vi "stations Template Keys.vi"(7 "Station ID (\"\")":string, 8 "error in (no error)":errorcluster, 9 "Copy? (f)":bool, 10 "Edit? (f)":bool, 11 "Connection Refnum":T1) -> (0 "error out":errorcluster, 1 "Template Keys":T2, 3 "Connection Refnum":T1)   [LabVIEW 2011]
uses:
  ITK EXT/utils/keyedarr.llb/Keyed Array.ctl
  Summitek EXT/ODBC/SQL Controls/Connection Refnum.ctl
  server/database/Drivers/Driver Table Fields.ctl
  ITK EXT/utils/strutil.llb/Case Matching.ctl
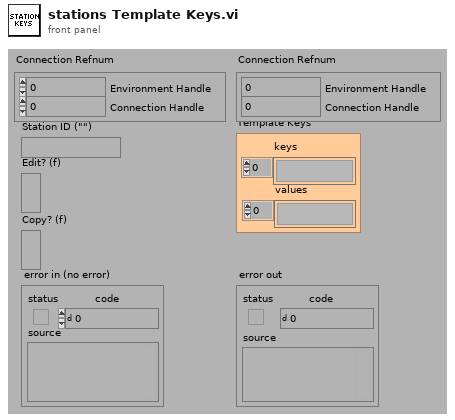
[diagram p1: front panel]
types:
  T1 = typedef "Connection Refnum.ctl" = cluster{"Environment Handle":i32, "Connection Handle":i32}
  T2 = typedef "Keyed Array.ctl" = cluster{"keys":string[], "values":string[]}
  T3 = typedef "Driver Table Fields.ctl" = enum16{"sxDriverId", "sType", "sVersion", "ixDriver"}
  T4 = typedef "Instrument Record.ctl" = cluster{"ixInstrument":i32, "sxInstrumentId":string, "sDriverId":string, "sDriverType":string, "sSerialNumber":string, "tLastCalibration":timestamp, "tCalibrationDue":timestamp, "sConfiguration":string}
  T5 = typedef "Station Record.ctl" = cluster{"ixStation":i32, "sxStationId":string, "sIP":string, "fVerified":bool}
  T6 = typedef "Driver Record.ctl" = cluster{"ixDriver":i32, "sxDriverId":string, "sType":string, "sVersion":string}
  T7 = typedef "Case Matching.ctl" = enum16{"a != A", "a == A", "system"}
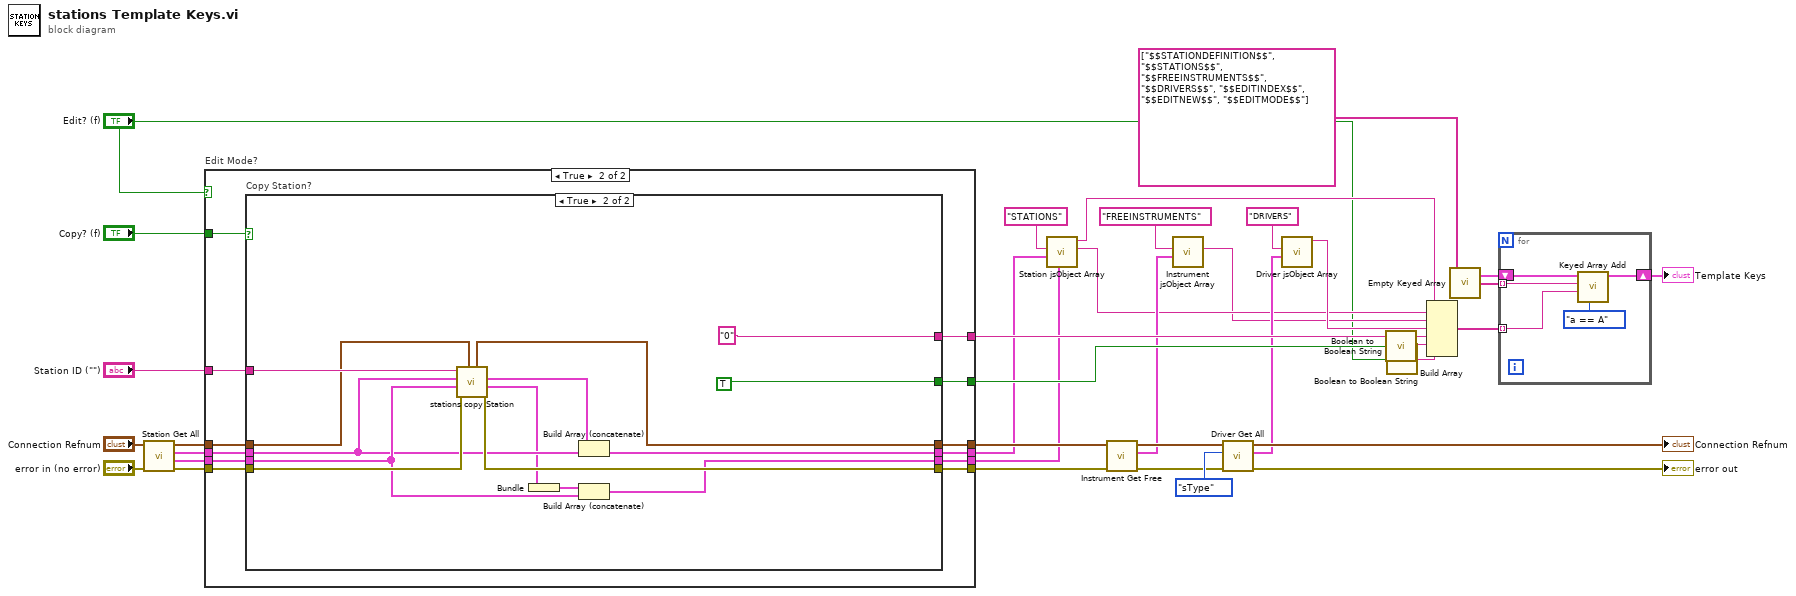
[diagram p0: block diagram]
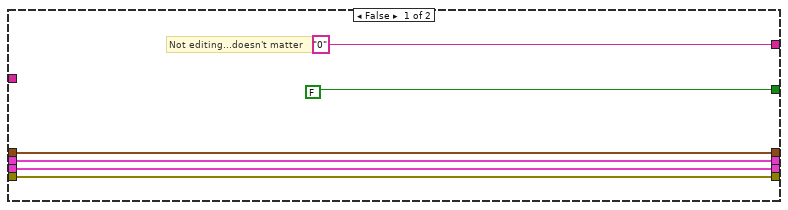
[diagram p2: hidden frame]
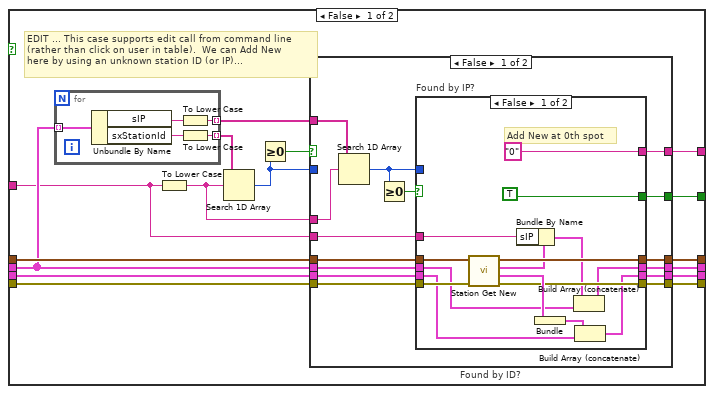
[diagram p3: hidden frame]
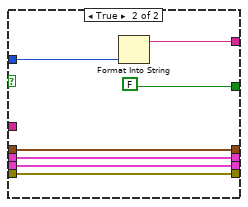
[diagram p4: hidden frame]
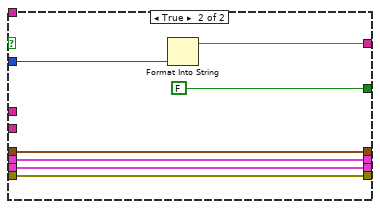
[diagram p5: hidden frame]
diagram:
  n1 = call "Station Get All.vi"("error in (no error)"="error in (no error)", "Connection Refnum"="Connection Refnum") -> ("error out"=w27:errorcluster, "All Station Instruments"=w22:cluster{"Instruments":T4[]}[], "Station Records"=w23:T5[], "Connection Refnum"=w24:T1)  [unwired: 2 in, 4 out]
  n2 = case "Edit Mode?" shown="True" "Edit? (f)" {
    tunnel: w23 -> [w41 w53]
    tunnel: [w41 w42] -> w13
    tunnel: w27 -> [w40 w52]
    tunnel: [w40 w51] -> w17
    tunnel: ["0" w50] -> w21
    tunnel: "Station ID (\"\")" -> [_ w49]
    tunnel: [FALSE w48] -> w19
    tunnel: "Copy? (f)" -> [_ w47]
    tunnel: w24 -> [w37 w44]
    tunnel: w22 -> [w38 w46]
    tunnel: [w38 w45] -> w12
    tunnel: [w37 w43] -> w15
    frame False {
      # "Not editing...doesn't matter"
    }
    frame True {
      n3 = case "Copy Station?" shown="True" w47 {
        tunnel: w49 -> [w54 w127]
        tunnel: w53 -> [w58 w123]
        tunnel: [w67 "0"] -> w50
        tunnel: [w66 w129] -> w51
        tunnel: w52 -> [w65 w130]
        tunnel: [w64 TRUE] -> w48
        tunnel: [w56 w128] -> w42
        tunnel: w46 -> [w57 w126]
        tunnel: [w55 w121] -> w45
        tunnel: w44 -> [w60 w120]
        tunnel: [w59 w119] -> w43
        frame False {
          # "EDIT ... This case supports edit call from command line\n(rather than click on user in table).  We can Add New\nhere by using an unknown station ID (or IP)..."
          n4 = for {
            tunnel: [w118] -> w69 mode=indexing
            tunnel: w58 -> [w117] mode=indexing
            tunnel: [w114] -> w62 mode=indexing
            n5 = Unbundle By Name(w117) -> ("sIP"=w115:string, "sxStationId"=w116:string)
            n6 = To Lower Case(string=w115) -> (all lower case string=w114:string)
            n7 = To Lower Case(string=w116) -> (all lower case string=w118:string)
          }
          n8 = To Lower Case(string=w54) -> (all lower case string=w61:string)
          n9 = Search 1D Array(1D array=w69, element=w61) -> (index of element=w68:i32)  [unwired: 1 out]
          n10 = Greater Or Equal To 0?(x=w68) -> (x >= 0?=w63:bool)
          n11 = case "Found by ID?" shown="False" w63 {
            tunnel: w68 -> [_ w113]
            tunnel: [w81 w112] -> w67
            tunnel: [w76 w110] -> w66
            tunnel: w65 -> [w77 w110]
            tunnel: [w80 FALSE] -> w64
            tunnel: w62 -> [w84 _]
            tunnel: w61 -> [w83 _]
            tunnel: w60 -> [w79 w109]
            tunnel: [w78 w109] -> w59
            tunnel: w58 -> [w75 w108]
            tunnel: w57 -> [w73 w107]
            tunnel: [w74 w108] -> w56
            tunnel: [w72 w107] -> w55
            tunnel: w54 -> [w70 _]
            frame False {
              n12 = Search 1D Array(1D array=w84, element=w83) -> (index of element=w82:i32)  [unwired: 1 out]
              n13 = Greater Or Equal To 0?(x=w82) -> (x >= 0?=w71:bool)
              n14 = case "Found by IP?" shown="False" w71 {
                tunnel: w82 -> [_ w106]
                tunnel: ["0" w105] -> w81
                tunnel: [TRUE FALSE] -> w80
                tunnel: w79 -> [w95 w103]
                tunnel: [w92 w103] -> w78
                tunnel: [w93 w102] -> w76
                tunnel: w77 -> [w94 w102]
                tunnel: [w89 w101] -> w74
                tunnel: w75 -> [w91 w101]
                tunnel: w73 -> [w90 w100]
                tunnel: [w88 w100] -> w72
                tunnel: w70 -> [w85 _]
                frame False {
                  # "Add New at 0th spot"
                  n15 = call "Station Get New.vi"("error in (no error)"=w94, "Connection Refnum"=w95) -> ("error out"=w93:errorcluster, "Instruments on Station"=w96:T4[], "New Test Station"=w87:T5, "Connection Refnum"=w92:T1)  [unwired: 6 out]
                  n16 = Bundle By Name(cluster=w87, "sIP"=w85) -> (w86:T5)
                  n17 = Bundle("Instruments on Station"=w96) -> (w97:cluster{"Instruments on Station":T4[]})  [unwired: 1 in]
                  n18 = Build Array (concatenate)(w86, w91) -> (w89:T5[])
                  n19 = Build Array (concatenate)(w97, w90) -> (w88:cluster{"Instruments":T4[]}[])
                }
                frame True {
                  n20 = Format Into String(w106) -> (resulting string=w105:string)  [unwired: 3 in, 1 out]
                }
              }
            }
            frame True {
              n21 = Format Into String(w113) -> (resulting string=w112:string)  [unwired: 3 in, 1 out]
            }
          }
        }
        frame True {
          n22 = call "stations copy Station.vi"("Connection Refnum"=w120, "error in (no error)"=w130, "Stations Instruments"=w126, "All Stations (empty)"=w123, "Station ID to Copy (\"\")"=w127) -> ("error out"=w129:errorcluster, "Station Instruments"=w122:T4[], "Station Record"=w124:T5, "Connection Refnum"=w119:T1)  [unwired: 3 out]
          n23 = Bundle("Station Instruments"=w122) -> (w125:cluster{"Station Instruments":T4[]})  [unwired: 1 in]
          n24 = Build Array (concatenate)(w124, w123) -> (w128:T5[])
          n25 = Build Array (concatenate)(w125, w126) -> (w121:cluster{"Instruments":T4[]}[])
        }
      }
    }
  }
  n26 = call "Station jsObject Array.vi"("Stations Instruments (none)"=w12, "Stations (empty)"=w13, "Stations jsObject Array Name (\"STATIONS\")"="STATIONS" ("Stations jsObject Array Name (\"\")")) -> ("Stations jsObject Array"=w4:string, "Station jsObject Definition"=w3:string)  [unwired: 2 in, 5 out]
  n27 = call "Instrument Get Free.vi"("error in (no error)"=w17, "Connection Refnum"=w15) -> ("error out"=w18:errorcluster, "Free Instruments"=w10:T4[], "Connection Refnum"=w16:T1)  [unwired: 3 out]
  n28 = call "Instrument jsObject Array.vi"("Instruments (empty)"=w10, "Instruments jsObject Array Name (\"INSTRUMENTS\")"="FREEINSTRUMENTS" ("Stations jsObject Array Name (\"\")")) -> ("Instruments jsObject Array"=w2:string)  [unwired: 2 in, 7 out]
  n29 = call "Driver Get All.vi"("error in (no error)"=w18, "Sort by (sxDriverId)"=Driver_Table_Fields."sType" ("Sort by (Driver_ID)"), "Connection Refnum"=w16) -> ("error out"=→"error out":errorcluster, "Drivers"=w6:T6[], "Connection Refnum"=→"Connection Refnum":T1)  [unwired: 1 in, 5 out]
  n30 = call "Driver jsObject Array.vi"("DRIVERS (empty)"=w6, "Drivers jsObject Array Name (\"\")"="DRIVERS" ("Drivers jsObject Array Name (\"\")")) -> ("Drivers jsObject Array"=w9:string)  [unwired: 3 in, 6 out]
  n31 = call "Boolean to Boolean String.vi"("Boolean"=w19) -> ("Boolean string"=w20:string)  [unwired: 1 in]
  n32 = call "Boolean to Boolean String.vi"("Boolean"="Edit? (f)") -> ("Boolean string"=w5:string)  [unwired: 1 in]
  n33 = Build Array(w3, w4, w2, w9, w21, w20, w5) -> (w32:string[])
  n34 = call "Empty Keyed Array.vi"() -> ("empty keyed array"=w35:T2)  [unwired: 3 out]
  n35 = for {
    shift-right: [w134] -> w33
    shift-left: w35 -> [w136]
    tunnel: string[] ["$$STATIONDEFINITION$$", "$$STATIONS$$", "$$FREEINSTRUMENTS$$", "$$DRIVERS$$", "$$EDITINDEX$$", "$$EDITNEW$$", "$$EDITMODE$$"] -> [w135] mode=indexing
    tunnel: w32 -> [w133] mode=indexing
    n36 = call "Keyed Array Add.vi"("case matching (sensitive)"=Case_Matching."a == A", "value"=w133, "key"=w135, "array in"=w136) -> ("array out"=w134:T2)  [unwired: 3 out]
  }
  "Template Keys" <- w33
